vi "Status.vi"(5 "Membrane washing status":bool, 7 "Column washing status":bool, 8 "Membrane washing error":bool, 9 "Bioreactor error":bool, 10 "Column washing error":bool, 11 "Error input":bool, 12 "2 step error":bool, 13 "2 step error-1":bool, 14 "2 step error-2":bool, 15 "1 step error":bool) -> (2 "Status output":string)   [LabVIEW 2019]
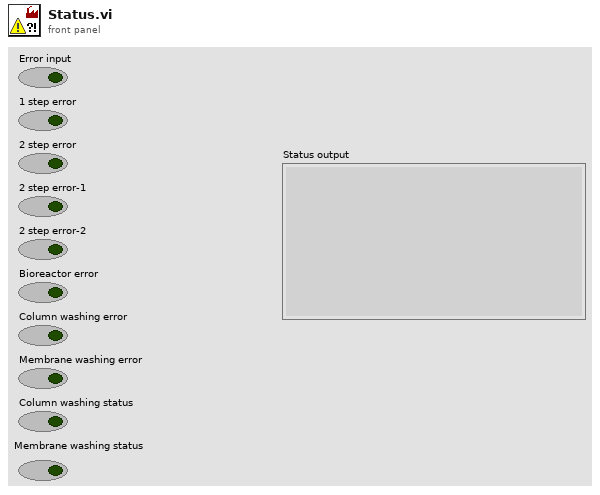
[diagram p1: front panel]
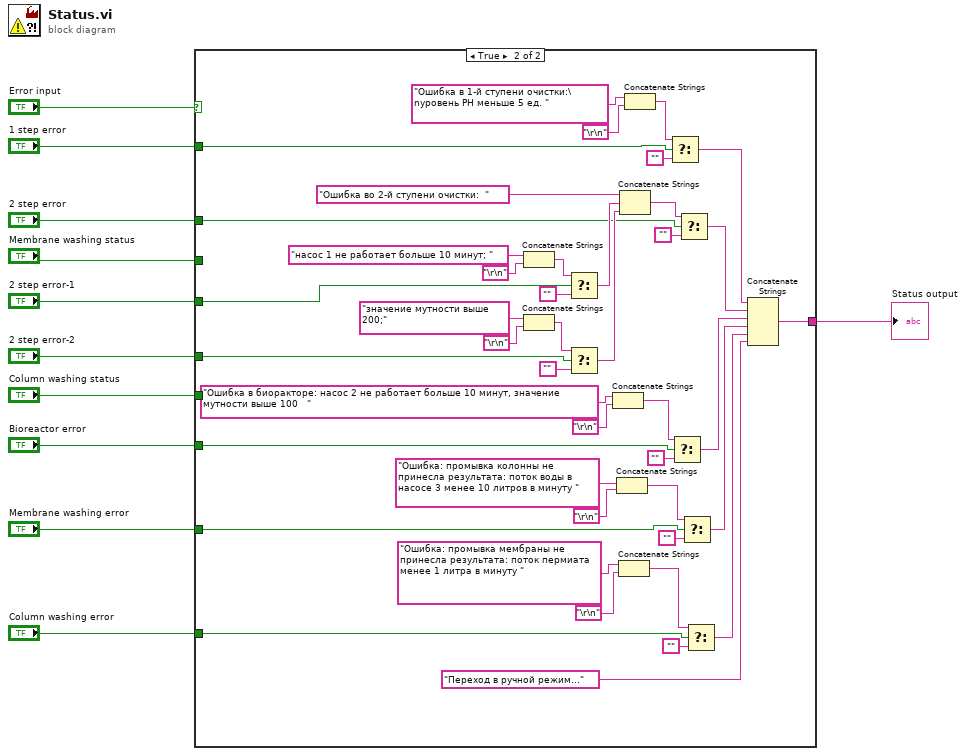
[diagram p0: block diagram]
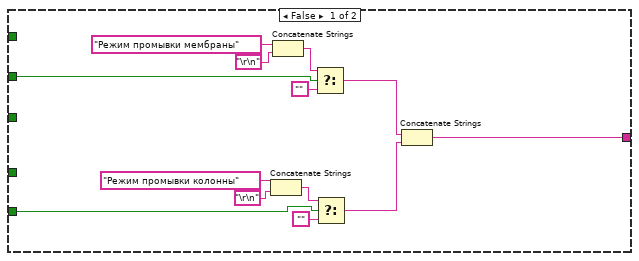
[diagram p2: hidden frame]
diagram:
  n1 = case shown="True" "Error input" {
    tunnel: "Bioreactor error" -> [_ w49]
    tunnel: "Column washing error" -> [_ w47]
    tunnel: "Membrane washing error" -> [_ w43]
    tunnel: "2 step error-2" -> [_ w41]
    tunnel: "2 step error-1" -> [_ w37]
    tunnel: "2 step error" -> [_ w32]
    tunnel: "1 step error" -> [_ w30]
    tunnel: [w12 w25] -> w11
    tunnel: "Membrane washing status" -> [w16 _]
    tunnel: "Column washing status" -> [w15 _]
    frame False {
      n2 = Concatenate Strings("Режим промывки колонны", "\r\n") -> (w19:string)
      n3 = Concatenate Strings("Режим промывки мембраны", "\r\n") -> (w17:string)
      n4 = Select(t=w17, s=w16, f="") -> (s? t:f=w14:string)
      n5 = Select(t=w19, s=w15, f="") -> (s? t:f=w13:string)
      n6 = Concatenate Strings(w14, w13) -> (w12:string)
    }
    frame True {
      n7 = Concatenate Strings("насос 1 не работает больше 10 минут; ", "\r\n") -> (w56:string)
      n8 = Concatenate Strings("значение мутности выше 200;", "\r\n") -> (w57:string)
      n9 = Select(t=w56, s=w37, f="") -> (s? t:f=w58:string)
      n10 = Select(t=w57, s=w41, f="") -> (s? t:f=w59:string)
      n11 = Concatenate Strings("Ошибка в биоракторе: насос 2 не работает больше 10 минут, значение мутности выше 100   ", "\r\n") -> (w62:string)
      n12 = Concatenate Strings("Ошибка: промывка колонны не принесла результата: поток воды в насосе 3 менее 10 литров в минуту ", "\r\n") -> (w60:string)
      n13 = Concatenate Strings("Ошибка: промывка мембраны не принесла результата: поток пермиата менее 1 литра в минуту ", "\r\n") -> (w61:string)
      n14 = Concatenate Strings("Ошибка во 2-й ступени очистки:  ", w58, w59) -> (w55:string)
      n15 = Concatenate Strings("Ошибка в 1-й ступени очистки:\nуровень PH меньше 5 ед. ", "\r\n") -> (w54:string)
      n16 = Select(t=w54, s=w30, f="") -> (s? t:f=w63:string)
      n17 = Select(t=w62, s=w49, f="") -> (s? t:f=w65:string)
      n18 = Select(t=w55, s=w32, f="") -> (s? t:f=w64:string)
      n19 = Select(t=w60, s=w43, f="") -> (s? t:f=w66:string)
      n20 = Select(t=w61, s=w47, f="") -> (s? t:f=w67:string)
      n21 = Concatenate Strings(w63, w64, w65, w66, w67, "Переход в ручной режим...") -> (w25:string)
    }
  }
  "Status output" <- w11
